vi "Begin.vi"(8 "error in":errorcluster) -> (0 "error out":errorcluster)   [LabVIEW 2015]
doc: "Called before other user functions, this VI is expected to open initial I/O refnums, load in file data, and do all program initialization. Notice that the <B>error out</B> terminal is simply used for data flow. Wiring it to other structures or subVIs ensures that this VI runs first."
uses:
  <vilib>/Rock Robotics/SystemInterfaces/DIO/FPGA_DIOPWMChannel.ctl
  <vilib>/Rock Robotics/WPI/SafetyOutput/WPI_SafetyOutputConfigMenu.ctl
  <vilib>/Rock Robotics/WPI/DriverStation/WPI_DriverStationRobotMode2.ctl
  <vilib>/Rock Robotics/WPI/Joystick/WPI_JoystickDeviceEnum.ctl
  <vilib>/Rock Robotics/SystemInterfaces/DIO/FPGA_DIOChannel.ctl
  <vilib>/Rock Robotics/SystemInterfaces/AI/FPGA_AIChannel.ctl
  <vilib>/Rock Robotics/WPI/CAN/TalonSRX/WPI_CANTalonSRX_APIControlMode.ctl
  <vilib>/Rock Robotics/WPI/CAN/TalonSRX/WPI_CANTalonSRX_APIFeedbackSelect.ctl
  <vilib>/Rock Robotics/SystemInterfaces/AI/FPGA_AIGyroChannel.ctl
  <vilib>/Rock Robotics/SystemInterfaces/DIO/FPGA_DIORelayChannel.ctl
  <vilib>/Rock Robotics/WPI/Relay/WPI_RelayDirection.ctl
  <vilib>/Rock Robotics/WPI/RobotDrive/WPI_RobotDriveOpen2MotorWithVictor.vi
  Robot Global Data.vi
  <vilib>/Rock Robotics/WPI/MotorControl/WPI_MotorControlOpen VictorSP.vi
  <vilib>/Rock Robotics/WPI/Counter/WPI_CounterDigitalInputToDigitalSource.vi
  <vilib>/Rock Robotics/WPI/MotorControl/WPI_MotorControlOpenCANTalonSRX.vi
  <vilib>/Rock Robotics/WPI/Ultrasonic/WPI_SonarMB1010AnalogOpen.vi
  <vilib>/Rock Robotics/WPI/Ultrasonic/WPI_SonarMB1010AnalogRefNum Registry Set.vi
  <vilib>/Rock Robotics/WPI/Gyro/WPI_GyroAnalogOpen.vi
  <vilib>/Rock Robotics/WPI/MotorControl/WPI_MotorControlOpen Victor.vi
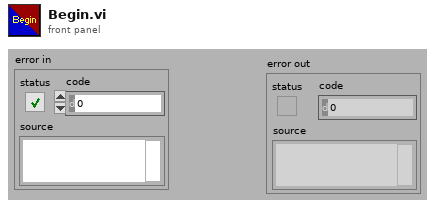
[diagram p1: front panel]
types:
  T1 = typedef "WPI_RelayDirection.ctl" = enum16{"Both directions", "Forward only", "Reverse only"}
  T2 = typedef "FPGA_DIORelayChannel.ctl" = enum8{"Relay 0", "Relay 1", "Relay 2", "Relay 3", "Invalid"}
  T3 = typedef "FPGA_DIOChannel.ctl" = enum8{"DIO 0", "DIO 1", "DIO 2", "DIO 3", "DIO 4", "DIO 5", "DIO 6", "DIO 7", "DIO 8", "DIO 9", "DIO MXP 0", "DIO MXP 1", "DIO MXP 2", "DIO MXP 3", "DIO MXP 4", "DIO MXP 5", "DIO MXP 6", "DIO MXP 7", "DIO MXP 8", "DIO MXP 9", "DIO MXP 10", "DIO MXP 11", "DIO MXP 12", "DIO MXP 13", "DIO MXP 14", "DIO MXP 15", "Invalid"}
  T4 = typedef "FPGA_DIOPWMChannel.ctl" = enum8{"PWM 0", "PWM 1", "PWM 2", "PWM 3", "PWM 4", "PWM 5", "PWM 6", "PWM 7", "PWM 8", "PWM 9", "PWM MXP 0", "PWM MXP 1", "PWM MXP 2", "PWM MXP 3", "PWM MXP 4", "PWM MXP 5", "PWM MXP 6", "PWM MXP 7", "PWM MXP 8", "PWM MXP 9", "Invalid"}
  T5 = typedef "WPI_JoystickDeviceEnum.ctl" = enum16{"USB 0", "USB 1", "USB 2", "USB 3", "USB 4", "USB 5"}
  T6 = typedef "WPI_CANTalonSRX_APIFeedbackSelect.ctl" = enum16{"Digital Quadrature Encoder", "Analog Potentiometer", "Analog Encoder", "Count on Quad-A (Rising-Edge)", "Count on Quad-A (Falling-Edge)", "CTR Magnetic Enc (Absolute)", "CTR Magnetic Enc (Relative)", "Pulse Width"}
  T7 = typedef "WPI_CANTalonSRX_APIControlMode.ctl" = enum8{"Percent VBus", "Speed", "Position", "Slave", "Unchanged / Invalid", "Voltage Compensation", "Current", "Motion Profile"}
  T8 = typedef "FPGA_AIGyroChannel.ctl" = enum8{"AI 0", "AI 1", "Invalid"}
  T9 = typedef "FPGA_AIChannel.ctl" = enum8{"AI 0", "AI 1", "AI 2", "AI 3", "AI MXP 0", "AI MXP 1", "AI MXP 2", "AI MXP 3", "Invalid"}
  T10 = typedef "WPI_DriverStationRobotMode2.ctl" = enum16{"Autonomous Disabled", "Autonomous Enabled", "Teleop Disabled", "Teleop Enabled", "Disconnected", "Finish", "Test Disabled", "Test Enabled", "Emergency Stopped"}
  T11 = typedef "WPI_SafetyOutputConfigMenu.ctl" = enum16{"Enable", "Disable"}
  T12 = typedef "WPI_MotorControlDeviceRef.ctl" = cluster{"DeviceStatus":errorcluster, "Type":T13, "PWM":cluster{"PWM Channel":T4, "DeadBand":T14}, "CAN":cluster{"Device Number":u8, "Control Mode":T15, "Semaphore":T16, "Max Vout":dbl, "TalonSRX Control Mode":T7}, "Invert":bool}
  T13 = typedef "WPI_MotorControlType.ctl" = enum16{"PWM", "CAN", "CANTalonSRX"}
  T14 = typedef "WPI_PWMDeadband.ctl" = cluster{"Name":string, "maxPositivePwm":i32, "minPositivePwm":i32, "centerPwm":i32, "maxNegativePwm":i32, "minNegativePwm":i32, "angularRange":u16}
  T15 = typedef "WPI_CANJaguar_ControlMode.ctl" = enum8{"Percent VBus", "Current", "Speed", "Position", "Voltage"}
  T16 = typedef "Semaphore RefNum" = refnum<k1>
  T17 = typedef "WPI_CANTalonSRX_GlobalStatus.ctl" = cluster{"Applied Throttle":dbl, "Module Enabled":bool, "CAN Error":errorcluster, "Closed Loop Error":dbl, "Forward Limit Switch Closed":bool, "Reverse Limit Switch Closed":bool, "Sensor Position":dbl, "Sensor Velocity":dbl, "Current":dbl, "Sticky Fault - Over Temp":bool, "Sticky Fault - Under Voltage":bool, "Sticky Fault - Forward Limit":bool, "Sticky Fault - Reverse Limit":bool, "Sticky Fault - Forward Soft Limit":bool, "Sticky Fault - Reverse Soft Limit":bool, "Brake is Enabled":bool, "Encoder Position":dbl, "Encoder Velocity":dbl, "Encoder Index Count":dbl, "Encoder A Pin State":bool, "Encoder B Pin State":bool, "Encoder Index Pin State":bool, "Analog In":dbl, "Analog In Velocity":dbl, "Temperature (C)":dbl, "Battery Voltage":dbl, "Control 5 Is Supported":bool, "Current Profile Slot Select":dbl, "Pos Div 8":bool, "Vel Div 4":bool, "Pulse Width Position":i32, "Pulse Width Velocity":i32, "Pulse Width Rise To Rise (us)":i32, "Pulse Width Rise To Fall (us)":i32, "Mot Prof Active Is Under Run":bool, "Mot Prof Active Has Under Run":bool, "Mot Prof Active Is Last":bool, "Mot Prof Active Velocity Only":bool, "Mot Prof Active Is Valid":bool, "Mot Prof Buffer Is Full":bool, "Mot Prof Active Profile Slot Select":i32, "Mot Prof NextID":i32, "Mot Prof Count":i32, "Mot Prof Active Velocity":dbl, "Mot Prof Active Position":dbl, "Mot Prof Output Enable":i32}
  T18 = typedef "WPI_DigitalInputDevRef.ctl" = cluster{"DevStatus":errorcluster, "DIO Channel":T3}
  T19 = typedef "WPI_RelayDevRef.ctl" = cluster{"DevStatus":errorcluster, "Relay Channel":T2, "Relay Direction":T1}
  T20 = typedef "WPI_GyroDevRef.ctl" = cluster{"DevStatus":errorcluster, "Analog Channel":T9, "Offset":dbl, "Gain (VoltsPerDegree/Second)":dbl, "Gyro Type":enum16{"Analog", "XRS450"}, "Handle":i32, "SPI Bus":T21, "Device Found":bool, "Sample Rate":dbl, "Calibrate On Open":bool}
  T21 = typedef "spi_bus.ctl" = enum16{"SPI On-Board, CS0", "SPI On-Board, CS1", "SPI On-Board, CS2", "SPI On-Board, CS3", "SPI MXP", "Invalid"}
  T22 = typedef "WPI_JoystickDevRef.ctl" = cluster{"Device":T5}
  T23 = typedef "FPGA_CounterEncoderSourceConvertionLVSourceType.ctl" = cluster{"DevStatus":errorcluster, "AnalogTriggerMode?":bool, "DigitalMode":cluster{"DIO Channel":T24}, "AnalogTriggerMode":cluster{"AnalogTriggerIndex":T25, "OutputType":T26}}
  T24 = typedef "FPGA_DIODigitalSourceChannel.ctl" = enum8{"DIO 0", "DIO 1", "DIO 2", "DIO 3", "DIO 4", "DIO 5", "DIO 6", "DIO 7", "DIO 8", "DIO 9", "DIO MXP 0", "DIO MXP 1", "DIO MXP 2", "DIO MXP 3", "DIO MXP 4", "DIO MXP 5", "DIO MXP 6", "DIO MXP 7", "DIO MXP 8", "DIO MXP 9", "DIO MXP 10", "DIO MXP 11", "DIO MXP 12", "DIO MXP 13", "DIO MXP 14", "DIO MXP 15", "Disabled"}
  T25 = typedef "FPGA_AnalogTriggerIndex.ctl" = enum8{"Trig 0", "Trig 1", "Trig 2", "Trig 3", "Trig 4", "Trig 5", "Trig 6", "Trig 7", "Invalid"}
  T26 = typedef "FPGA_AnalogTriggerOutType.ctl" = enum16{"InWindow", "TriggerState", "Rising", "Falling"}
  T27 = typedef "WPI_SonarMB1010AnalogDeviceRef.ctl" = cluster{"AIDeviceRef":T28, "Scaling factor (V/in)":dbl, "Average Bits":u8}
  T28 = typedef "WPI_AnalogChannelDevRef.ctl" = cluster{"DevStatus":errorcluster, "Analog Channel":T9}
  T29 = typedef "WPI_EncoderDevRef.ctl" = cluster{"DevStatus":errorcluster, "EncoderIndex":T30, "CounterIndex":T31, "DistancePerCount":dbl, "Decoding Type":T32}
  T30 = typedef "FPGA_EncoderIdx.ctl" = enum8{"Enc 0", "Enc 1", "Enc 2", "Enc 3", "Enc 4", "Enc 5", "Enc 6", "Enc 7", "Invalid"}
  T31 = typedef "FPGA_CounterCtrSystemIndex.ctl" = enum8{"Ctr 0", "Ctr 1", "Ctr 2", "Ctr 3", "Ctr 4", "Ctr 5", "Ctr 6", "Ctr 7", "Invalid"}
  T32 = typedef "WPI_EncoderType.ctl" = enum16{"1x", "2x", "4x"}
  T33 = typedef "WPI_RobotDriveDevRef.ctl" = cluster{"DevStatus":errorcluster, "Motors[]":T12[], "Square Inputs":bool, "Max Output":dbl}
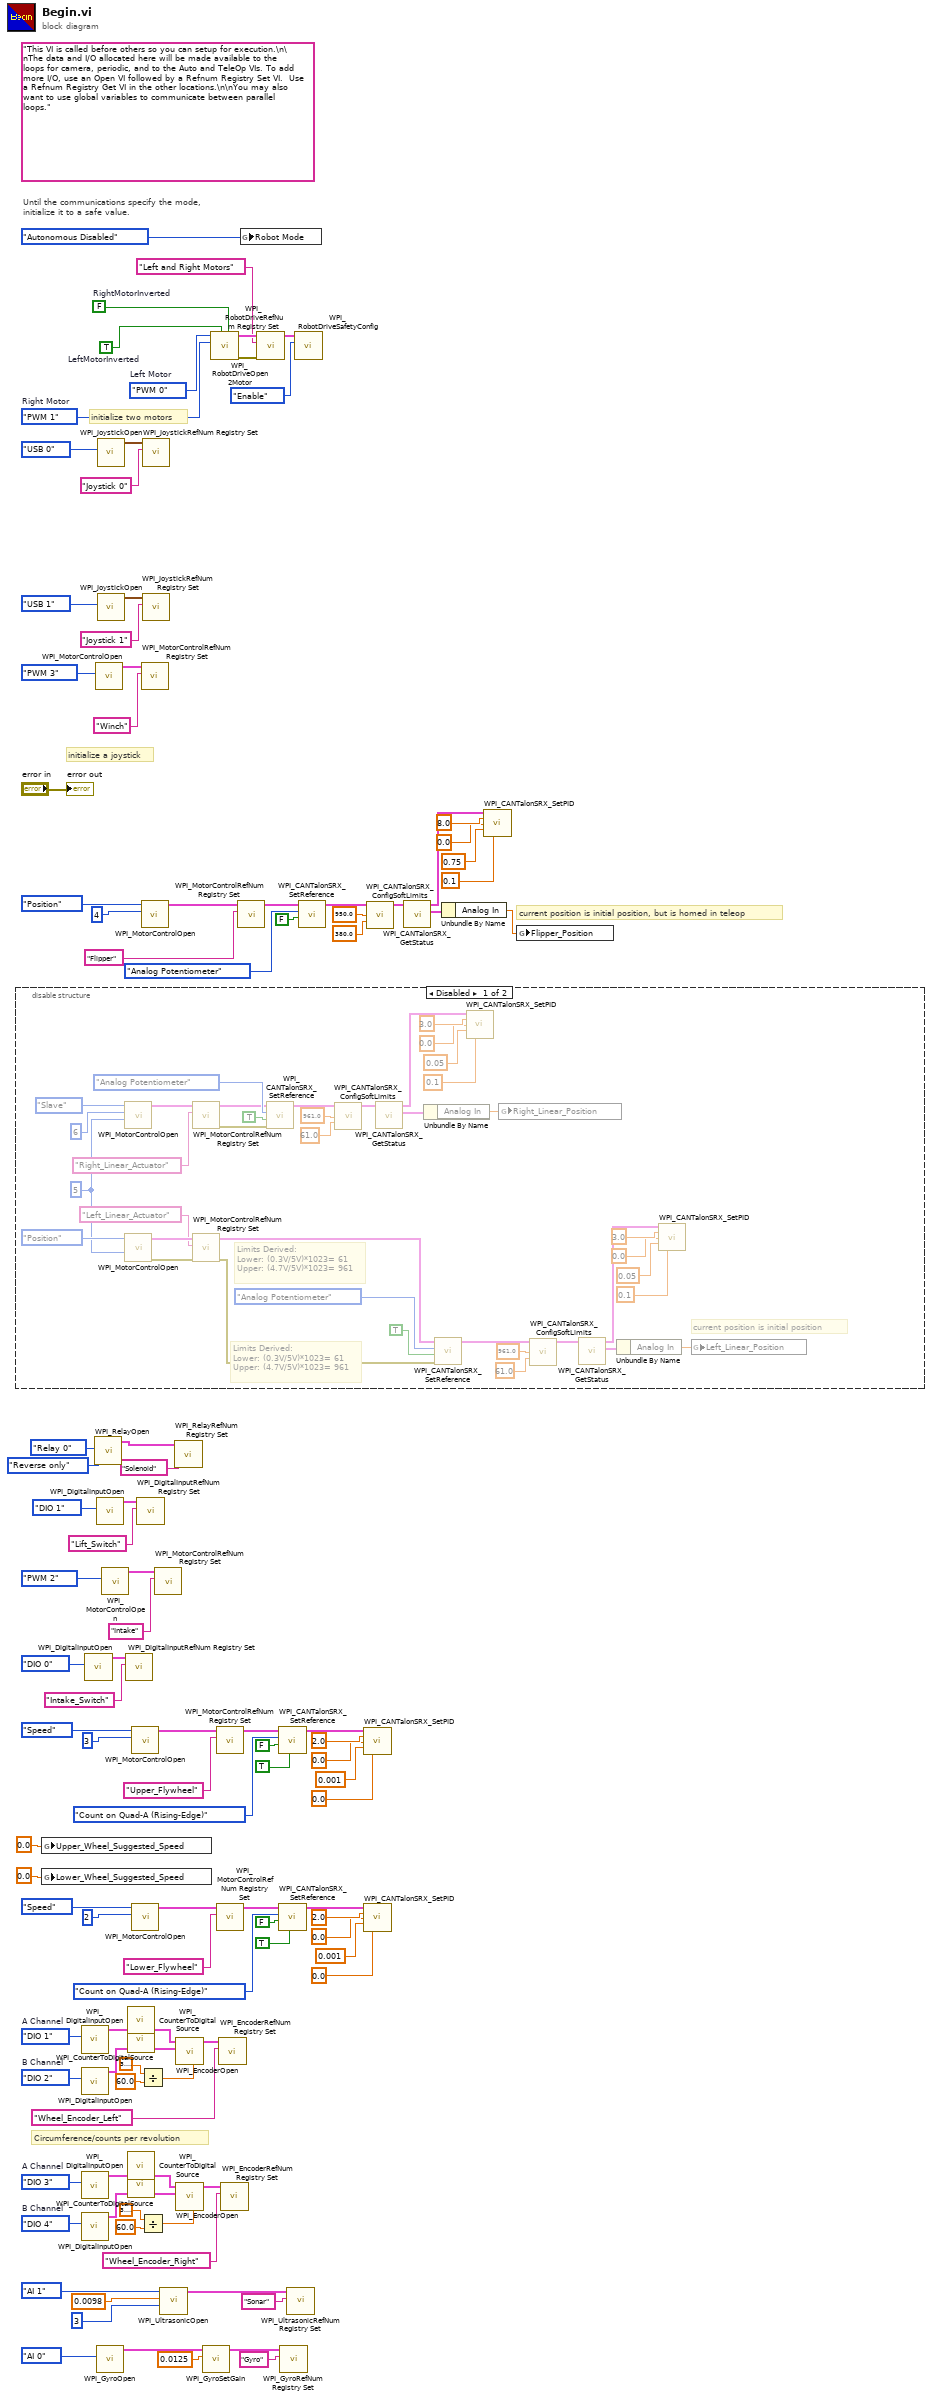
[diagram p0: block diagram]
diagram:
  w79 = FPGA_DIOChannel."DIO 4"  # B Channel
  w78 = FPGA_DIOChannel."DIO 3"  # A Channel
  w87 = FPGA_DIOChannel."DIO 2"  # B Channel
  w86 = FPGA_DIOChannel."DIO 1"  # A Channel
  (unwired) "This VI is called before others so you can setup for execution.\n\nThe data and I/O allocated here will be made available to the loops for camera, periodic, and to the Auto and TeleOp VIs. To add more I/O, use an Open VI followed by a Refnum Registry Set VI.  Use a Refnum Registry Get VI in the other locations.\n\nYou may also want to use global variables to communicate between parallel loops."
  w105 = FPGA_DIOPWMChannel."PWM 1"  # Right Motor
  w106 = FPGA_DIOPWMChannel."PWM 0"  # Left Motor
  w110 = TRUE  # LeftMotorInverted
  w111 = FALSE  # RightMotorInverted
  # "current position is initial position, but is homed in teleop"
  # "Circumference/counts per revolution"
  # "initialize a joystick"
  # "Until the communications specify the mode,\ninitialize it to a safe value."
  # "initialize two motors"
  n1 = disable-structure shown="Disabled" {
    frame Disabled {
      w144 = u8 5 ("Master Device Number")
      # "current position is initial position"
      # "Limits Derived: \nLower: (0.3V/5V)*1023= 61\nUpper: (4.7V/5V)*1023= 961"
      # "Limits Derived: \nLower: (0.3V/5V)*1023= 61\nUpper: (4.7V/5V)*1023= 961"
      n2 = call-poly <vilib>:"WPI_MotorControlOpen.vi"("Master Device Number"=w144, "Device Number"=u8 6, "Control Mode"=WPI_CANTalonSRX_APIControlMode."Slave") -> ("MotorControlDeviceRef"=w147:T12)  [unwired: 7 in, 1 out]
      n3 = call-poly <vilib>:"WPI_MotorControlOpen.vi"("Master Device Number"=w144, "Control Mode"=WPI_CANTalonSRX_APIControlMode."Position") -> ("error out"=w130:errorcluster, "MotorControlDeviceRef"=w150:T12)  [unwired: 8 in]
      n4 = call <vilib>:"WPI_MotorControlRefNum Registry Set.vi"("refnum name"="Right_Linear_Actuator", "MotorControlDevRef"=w147) -> ("error out"=w114:errorcluster, "MotorControlDevRef"=w115:T12)  [unwired: 8 in]
      n5 = call <vilib>:"WPI_MotorControlRefNum Registry Set.vi"("error in (no error)"=w130, "refnum name"="Left_Linear_Actuator", "MotorControlDevRef"=w150) -> ("error out"=w129:errorcluster, "MotorControlDevRef"=w131:T12)  [unwired: 7 in]
      n6 = call <vilib>:"WPI_CANTalonSRX_SetReference.vi"("error in (no error)"=w114, "Reverse Feedback Sensor"=TRUE, "Feedback Reference"=WPI_CANTalonSRX_APIFeedbackSelect."Analog Potentiometer", "CAN Talon SRX Ref"=w115) -> ("CAN Talon SRX Ref"=w125:T12)  [unwired: 6 in, 1 out]
      n7 = call <vilib>:"WPI_CANTalonSRX_ConfigSoftLimits.vi"("CAN Talon SRX Ref"=w125, "Forward Limit Position"=961.0, "Reverse Limit Position"=61.0) -> ("CAN Talon SRX Ref"=w126:T12)  [unwired: 11 in, 1 out]
      n8 = call <vilib>:"WPI_CANTalonSRX_GetStatus.vi"("CAN Talon SRX Ref"=w126) -> ("Talon SRX Status"=w127:T17, "CAN Talon SRX Ref"=w122:T12)  [unwired: 8 in, 1 out]
      n9 = Unbundle By Name(w127) -> ("Analog In"=w113:dbl)
      n10 = call <vilib>:"WPI_CANTalonSRX_SetReference.vi"("error in (no error)"=w129, "Reverse Feedback Sensor"=TRUE, "Feedback Reference"=WPI_CANTalonSRX_APIFeedbackSelect."Analog Potentiometer", "CAN Talon SRX Ref"=w131) -> ("CAN Talon SRX Ref"=w140:T12)  [unwired: 6 in, 1 out]
      n11 = call <vilib>:"WPI_CANTalonSRX_SetPID.vi"("CAN Talon SRX Ref"=w122, "P"=3.0, "I"=0.0, "D"=0.05, "F"=0.1) -> ()  [unwired: 9 in, 2 out]
      n12 = global write "Robot Global Data.vi" "Right_Linear_Position"(w113) -> ()
      n13 = call <vilib>:"WPI_CANTalonSRX_ConfigSoftLimits.vi"("CAN Talon SRX Ref"=w140, "Forward Limit Position"=961.0, "Reverse Limit Position"=61.0) -> ("CAN Talon SRX Ref"=w141:T12)  [unwired: 11 in, 1 out]
      n14 = call <vilib>:"WPI_CANTalonSRX_GetStatus.vi"("CAN Talon SRX Ref"=w141) -> ("Talon SRX Status"=w142:T17, "CAN Talon SRX Ref"=w137:T12)  [unwired: 8 in, 1 out]
      n15 = Unbundle By Name(w142) -> ("Analog In"=w112:dbl)
      n16 = call <vilib>:"WPI_CANTalonSRX_SetPID.vi"("CAN Talon SRX Ref"=w137, "P"=3.0, "I"=0.0, "D"=0.05, "F"=0.1) -> ()  [unwired: 9 in, 2 out]
      n17 = global write "Robot Global Data.vi" "Left_Linear_Position"(w112) -> ()
    }
    frame Enabled {
    }
  }
  n18 = global write "Robot Global Data.vi" "Upper_Wheel_Suggested_Speed"(0.0 ("Upper_Wheel_Suggested_Speed")) -> ()
  n19 = global write "Robot Global Data.vi" "Lower_Wheel_Suggested_Speed"(0.0 ("Upper_Wheel_Suggested_Speed")) -> ()
  n20 = call <vilib>:"WPI_DigitalInputOpen.vi"("DIO Channel"=w86) -> ("DigitalInputDevRef"=w83:T18)  [unwired: 1 in, 9 out]
  n21 = call <vilib>:"WPI_DigitalInputOpen.vi"("DIO Channel"=w87) -> ("DigitalInputDevRef"=w84:T18)  [unwired: 1 in, 9 out]
  n22 = call <vilib>:"WPI_DigitalInputOpen.vi"("DIO Channel"=w78) -> ("DigitalInputDevRef"=w75:T18)  [unwired: 1 in, 9 out]
  n23 = call <vilib>:"WPI_DigitalInputOpen.vi"("DIO Channel"=w79) -> ("DigitalInputDevRef"=w76:T18)  [unwired: 1 in, 9 out]
  n24 = call <vilib>:"WPI_DigitalInputOpen.vi"("DIO Channel"=FPGA_DIOChannel."DIO 0") -> ("DigitalInputDevRef"=w93:T18)  [unwired: 1 in, 9 out]
  n25 = call <vilib>:"WPI_RelayOpen.vi"("Relay Direction"=WPI_RelayDirection."Reverse only", "Relay Channel"=FPGA_DIORelayChannel."Relay 0") -> ("RelayDevRef"=w2:T19)  [unwired: 8 in, 1 out]
  n26 = call-poly <vilib>:"WPI_MotorControlOpen.vi"("PWM Channel"=FPGA_DIOPWMChannel."PWM 3") -> ("MotorControlDeviceRef"=w10:T12)  [unwired: 9 in, 1 out]
  n27 = call <vilib>:"WPI_DigitalInputOpen.vi"("DIO Channel"=FPGA_DIOChannel."DIO 1") -> ("DigitalInputDevRef"=w6:T18)  [unwired: 1 in, 9 out]
  n28 = call-poly <vilib>:"WPI_GyroOpen.vi"("Analog Channel"=FPGA_AIGyroChannel."AI 0") -> ("GyroDevRef"=w41:T20)  [unwired: 8 in, 2 out]
  n29 = call <vilib>:"WPI_JoystickOpen.vi"("JoystickDevice"=WPI_JoystickDeviceEnum."USB 0") -> ("JoystickDevRef"=w100:T22)  [unwired: 10 in]
  n30 = call <vilib>:"WPI_JoystickOpen.vi"("JoystickDevice"=WPI_JoystickDeviceEnum."USB 1") -> ("JoystickDevRef"=w12:T22)  [unwired: 10 in]
  n31 = call-poly <vilib>:"WPI_MotorControlOpen.vi"("PWM Channel"=FPGA_DIOPWMChannel."PWM 2") -> ("MotorControlDeviceRef"=w96:T12)  [unwired: 9 in, 1 out]
  n32 = call <vilib>:"WPI_DigitalInputRefNum Registry Set.vi"("refnum name"="Intake_Switch", "DigitalInputDevRef"=w93) -> ()  [unwired: 8 in, 2 out]
  n33 = call-poly <vilib>:"WPI_CounterToDigitalSource.vi"("DigitalInputDevRef"=w83) -> ("Digital Source"=w82:T23)  [unwired: 6 out]
  n34 = call-poly <vilib>:"WPI_CounterToDigitalSource.vi"("DigitalInputDevRef"=w84) -> ("Digital Source"=w85:T23)  [unwired: 6 out]
  n35 = call-poly <vilib>:"WPI_CounterToDigitalSource.vi"("DigitalInputDevRef"=w75) -> ("Digital Source"=w74:T23)  [unwired: 6 out]
  n36 = call-poly <vilib>:"WPI_CounterToDigitalSource.vi"("DigitalInputDevRef"=w76) -> ("Digital Source"=w77:T23)  [unwired: 6 out]
  n37 = call-poly <vilib>:"WPI_MotorControlOpen.vi"("Device Number"=u8 3, "Control Mode"=WPI_CANTalonSRX_APIControlMode."Speed") -> ("MotorControlDeviceRef"=w91:T12)  [unwired: 8 in, 1 out]
  n38 = call-poly <vilib>:"WPI_MotorControlOpen.vi"("Device Number"=u8 2, "Control Mode"=WPI_CANTalonSRX_APIControlMode."Speed") -> ("MotorControlDeviceRef"=w89:T12)  [unwired: 8 in, 1 out]
  n39 = call <vilib>:"WPI_DigitalInputRefNum Registry Set.vi"("refnum name"="Lift_Switch", "DigitalInputDevRef"=w6) -> ()  [unwired: 8 in, 2 out]
  n40 = Divide(x=3.141592653589793, y=60.0 ("DistancePerCount")) -> (x/y=w47:dbl)
  n41 = Divide(x=3.141592653589793, y=60.0 ("DistancePerCount")) -> (x/y=w43:dbl)
  n42 = call <vilib>:"WPI_MotorControlRefNum Registry Set.vi"("refnum name"="Winch", "MotorControlDevRef"=w10) -> ()  [unwired: 8 in, 2 out]
  n43 = call-poly <vilib>:"WPI_MotorControlOpen.vi"("Device Number"=u8 4, "Control Mode"=WPI_CANTalonSRX_APIControlMode."Position") -> ("MotorControlDeviceRef"=w35:T12)  [unwired: 8 in, 1 out]
  n44 = call <vilib>:"WPI_JoystickRefNum Registry Set.vi"("refnum name"="Joystick 0", "JoystickDevRef"=w100) -> ()  [unwired: 8 in, 2 out]
  n45 = call <vilib>:"WPI_JoystickRefNum Registry Set.vi"("refnum name"="Joystick 1", "JoystickDevRef"=w12) -> ()  [unwired: 8 in, 2 out]
  n46 = call <vilib>:"WPI_MotorControlRefNum Registry Set.vi"("refnum name"="Intake", "MotorControlDevRef"=w96) -> ()  [unwired: 8 in, 2 out]
  n47 = call-poly <vilib>:"WPI_UltrasonicOpen.vi"("Average Bits"=u8 3, "Scaling factor (V/in)"=0.0098, "Analog Channel"=FPGA_AIChannel."AI 1") -> ("SonarMB1010AnalogDevRef"=w68:T27)  [unwired: 7 in, 1 out]
  n48 = call <vilib>:"WPI_RelayRefNum Registry Set.vi"("refnum name"="Solenoid", "RelayDevRef"=w2) -> ()  [unwired: 8 in, 2 out]
  n49 = call <vilib>:"WPI_EncoderOpen.vi"("DistancePerCount"=w47, "BSource"=w85, "ASource"=w82) -> ("EncoderDevRef"=w81:T29)  [unwired: 5 in, 3 out]
  n50 = call <vilib>:"WPI_EncoderOpen.vi"("DistancePerCount"=w43, "BSource"=w77, "ASource"=w74) -> ("EncoderDevRef"=w73:T29)  [unwired: 5 in, 3 out]
  n51 = call <vilib>:"WPI_GyroSetGain.vi"("Gain (VoltsPerDegree/Second)"=0.0125, "GyroDevRef"=w41) -> ("GyroDevRef"=w39:T20)  [unwired: 8 in, 1 out]
  n52 = call-poly <vilib>:"WPI_RobotDriveOpen2Motor.vi"("Right Motor Inverted"=w111, "Left Motor Inverted"=w110, "Right Motor"=w105, "Left Motor"=w106) -> ("error out"=w107:errorcluster, "RobotDriveDevRef"=w109:T33)  [unwired: 1 in, 5 out]
  n53 = call <vilib>:"WPI_MotorControlRefNum Registry Set.vi"("refnum name"="Upper_Flywheel", "MotorControlDevRef"=w91) -> ("MotorControlDevRef"=w64:T12)  [unwired: 8 in, 1 out]
  n54 = call <vilib>:"WPI_MotorControlRefNum Registry Set.vi"("refnum name"="Lower_Flywheel", "MotorControlDevRef"=w89) -> ("MotorControlDevRef"=w62:T12)  [unwired: 8 in, 1 out]
  n55 = call <vilib>:"WPI_EncoderRefNum Registry Set.vi"("refnum name"="Wheel_Encoder_Left", "EncoderDevRef"=w81) -> ()  [unwired: 8 in, 2 out]
  n56 = call <vilib>:"WPI_EncoderRefNum Registry Set.vi"("refnum name"="Wheel_Encoder_Right", "EncoderDevRef"=w73) -> ()  [unwired: 8 in, 2 out]
  n57 = call <vilib>:"WPI_MotorControlRefNum Registry Set.vi"("refnum name"="Flipper", "MotorControlDevRef"=w35) -> ("MotorControlDevRef"=w33:T12)  [unwired: 8 in, 1 out]
  n58 = global write "Robot Global Data.vi" "Robot Mode"(WPI_DriverStationRobotMode2."Autonomous Disabled" ("Robot Mode")) -> ()
  n59 = call <vilib>:"WPI_RobotDriveRefNum Registry Set.vi"("error in (no error)"=w107, "refnum name"="Left and Right Motors", "RobotDriveDevRef"=w109) -> ("RobotDriveDevRef"=w104:T33)  [unwired: 1 in, 7 out]
  n60 = call <vilib>:"WPI_CANTalonSRX_SetReference.vi"("Reverse Closed-Loop Output"=TRUE, "Reverse Feedback Sensor"=FALSE, "Feedback Reference"=WPI_CANTalonSRX_APIFeedbackSelect."Count on Quad-A (Rising-Edge)", "CAN Talon SRX Ref"=w64) -> ("CAN Talon SRX Ref"=w60:T12)  [unwired: 6 in, 1 out]
  n61 = call <vilib>:"WPI_CANTalonSRX_SetReference.vi"("Reverse Closed-Loop Output"=TRUE, "Reverse Feedback Sensor"=FALSE, "Feedback Reference"=WPI_CANTalonSRX_APIFeedbackSelect."Count on Quad-A (Rising-Edge)", "CAN Talon SRX Ref"=w62) -> ("CAN Talon SRX Ref"=w53:T12)  [unwired: 6 in, 1 out]
  n62 = call <vilib>:"WPI_GyroRefNum Registry Set.vi"("refnum name"="Gyro", "GyroDevRef"=w39) -> ()  [unwired: 8 in, 2 out]
  n63 = call-poly <vilib>:"WPI_UltrasonicRefNum Registry Set.vi"("refnum name"="Sonar", "SonarMB1010AnalogDevRef"=w68) -> ()  [unwired: 8 in, 2 out]
  n64 = call <vilib>:"WPI_RobotDriveSafetyConfig.vi"("mode"=WPI_SafetyOutputConfigMenu."Enable", "RobotDriveDevRef"=w104) -> ()  [unwired: 8 in, 2 out]
  n65 = call <vilib>:"WPI_CANTalonSRX_SetReference.vi"("Reverse Feedback Sensor"=FALSE, "Feedback Reference"=WPI_CANTalonSRX_APIFeedbackSelect."Analog Potentiometer", "CAN Talon SRX Ref"=w33) -> ("CAN Talon SRX Ref"=w29:T12)  [unwired: 7 in, 1 out]
  n66 = call <vilib>:"WPI_CANTalonSRX_SetPID.vi"("CAN Talon SRX Ref"=w60, "P"=2.0, "I"=0.0, "D"=0.001, "F"=0.0) -> ()  [unwired: 9 in, 2 out]
  n67 = call <vilib>:"WPI_CANTalonSRX_SetPID.vi"("CAN Talon SRX Ref"=w53, "P"=2.0, "I"=0.0, "D"=0.001, "F"=0.0) -> ()  [unwired: 9 in, 2 out]
  n68 = call <vilib>:"WPI_CANTalonSRX_ConfigSoftLimits.vi"("CAN Talon SRX Ref"=w29, "Forward Limit Position"=950.0, "Reverse Limit Position"=380.0) -> ("CAN Talon SRX Ref"=w30:T12)  [unwired: 11 in, 1 out]
  n69 = call <vilib>:"WPI_CANTalonSRX_GetStatus.vi"("CAN Talon SRX Ref"=w30) -> ("Talon SRX Status"=w31:T17, "CAN Talon SRX Ref"=w25:T12)  [unwired: 8 in, 1 out]
  n70 = Unbundle By Name(w31) -> ("Analog In"=w26:dbl)
  n71 = call <vilib>:"WPI_CANTalonSRX_SetPID.vi"("CAN Talon SRX Ref"=w25, "P"=8.0, "I"=0.0, "D"=0.75, "F"=0.1) -> ()  [unwired: 9 in, 2 out]
  n72 = global write "Robot Global Data.vi" "Flipper_Position"(w26) -> ()
  "error out" <- "error in"
